vi "啮合 扭矩最值.vi"(10 "扭矩正转":dbl[](array[numeric]), 11 "扭矩反转":dbl[](array[numeric])) -> (0 "反转最小值":dbl, 1 "反转最大值":dbl, 2 "正转最小值":dbl, 3 "正转最大值":dbl)   [LabVIEW 2015, in "Logging.lvlib"]
uses:
  Logging.lvlib
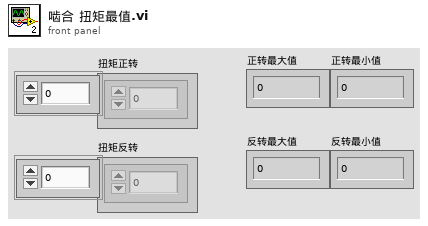
[diagram p1: front panel]
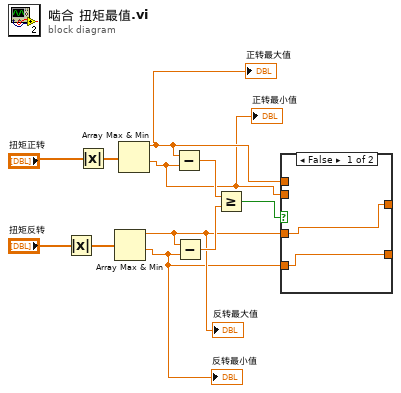
[diagram p0: block diagram]
diagram:
  n1 = Absolute Value(x="扭矩反转") -> (abs(x)=w7:dbl[])
  n2 = Absolute Value(x="扭矩正转") -> (abs(x)=w1:dbl[])
  n3 = Array Max & Min(array=w7) -> (max value=w4:dbl, min value=w3:dbl)  [unwired: 2 out]
  "反转最大值" <- w4
  "反转最小值" <- w3
  n4 = Array Max & Min(array=w1) -> (max value=w6:dbl, min value=w5:dbl)  [unwired: 2 out]
  "正转最大值" <- w6
  "正转最小值" <- w5
  n5 = Subtract(x=w6, y=w5) -> (x-y=w11:dbl)
  n6 = Subtract(x=w4, y=w3) -> (x-y=w10:dbl)
  n7 = Greater Or Equal?(x=w11, y=w10) -> (x >= y?=w9:bool)
  n8 = case shown="False" w9 {
    tunnel: w6 -> [_ w15]
    tunnel: [w13 w15] -> _
    tunnel: w5 -> [_ w14]
    tunnel: [w12 w14] -> _
    tunnel: w4 -> [w13 _]
    tunnel: w3 -> [w12 _]
    frame False {
    }
    frame True {
    }
  }
